vi "POIConvert.vi"(10 "POI array":dbl[][](array[numeric])) -> (3 "POISelectArrayOut":cluster{"System Array":dbl[], "Boolean":bool}[](array[cluster]))   [LabVIEW 2017]
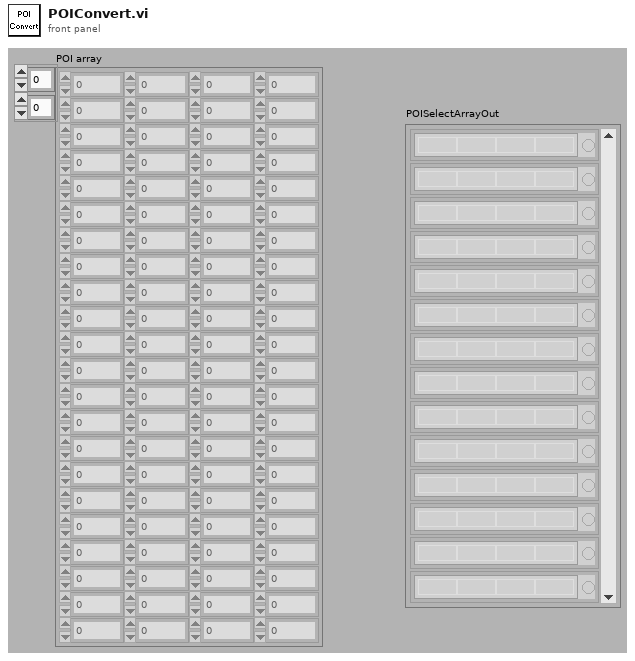
[diagram p1: front panel]
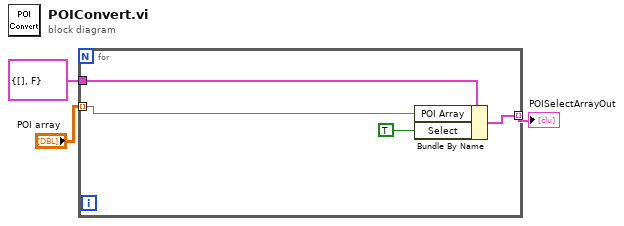
[diagram p0: block diagram]
diagram:
  n1 = for {
    tunnel: "POI array" -> [w6] mode=indexing
    tunnel: cluster{"POI Array":dbl[], "Select":bool} {"POI Array"=[], "Select"=FALSE} ("System Cluster") -> [w7]
    tunnel: [w5] -> w1 mode=indexing
    n2 = Bundle By Name(cluster=w7, "POI Array"=w6, "Select"=TRUE) -> (w5:cluster{"POI Array":dbl[], "Select":bool})
  }
  "POISelectArrayOut" <- w1
